vi "set_config_cluster.vi"(8 "error in (no error)":errorcluster, 10 "config cluster variant":variant, 11 "LightSourceDL090909Filament in":refnum<class "LightSourceDL090909Filament.lvclass">) -> (0 "error out":errorcluster, 3 "LightSourceDL090909Filament out":refnum<class "LightSourceDL090909Filament.lvclass">)   [LabVIEW 2010, in "LightSourceDL090909Filament.lvclass"]
uses:
  LightSourceDL090909Filament.lvclass
  LightSourceDL090909Filament.lvclass/LightSourceDL090909Filament.ctl
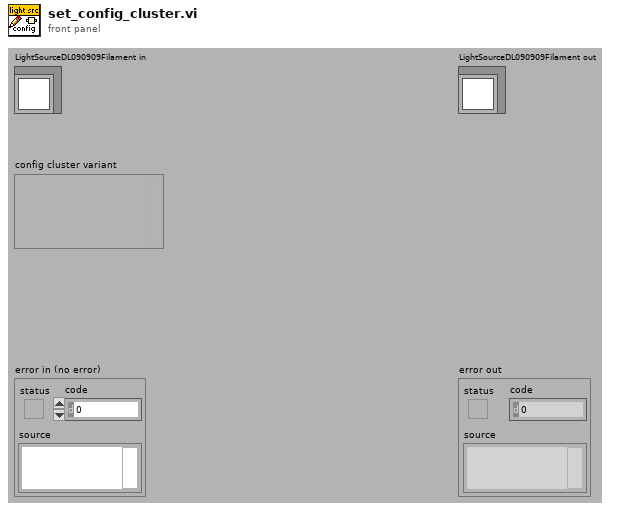
[diagram p1: front panel]
types:
  T1 = typedef "LightSourceDL090909Filament.lvclass/config_data_cluster.ctl" = cluster{"LSID":T2, "manufacturer specification":T3, "type":T4}
  T2 = typedef "LSID_cluster.ctl" = cluster{"identifier":string, "revision":i32}
  T3 = typedef "GenericComponent.lvclass/manufacturer_specification_cluster.ctl" = cluster{"manufacturer":string, "model":string, "serial number":string, "lot number":string}
  T4 = typedef "LightSourceDL090909Filament.lvclass/type_enum.ctl" = enum16{"Incandescent", "Halogen", "Unknown"}
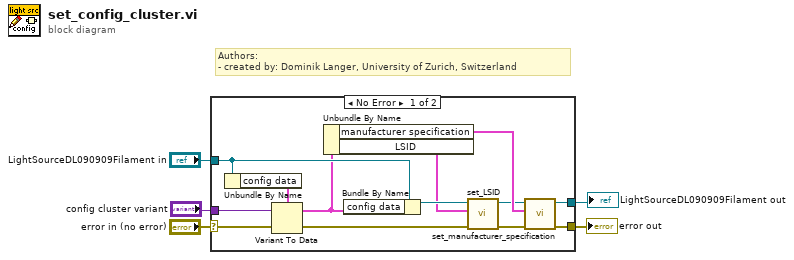
[diagram p0: block diagram]
diagram:
  # "Authors: \n- created by: Dominik Langer, University of Zurich, Switzerland"
  n1 = case shown="No Error" "error in (no error)" {
    selector: "error in (no error)" -> [w13 w20]
    tunnel: [w16 w20] -> w5
    tunnel: [w15 w19] -> w1
    tunnel: "LightSourceDL090909Filament in" -> [w12 w19]
    tunnel: "config cluster variant" -> [w14 _]
    frame No Error {
      n2 = Unbundle By Name(w12) -> ("config data"=w17:T1)
      n3 = Variant To Data(error in=w13, Variant=w14, type=w17) -> (error out=w18:errorcluster, data=w11:T1)
      n4 = Unbundle By Name(w11) -> ("manufacturer specification"=w8:T3, "LSID"=w9:T2)
      n5 = Bundle By Name(cluster=w12, "config data"=w11) -> (w10:refnum<class "LightSourceDL090909Filament.lvclass">)
      n6 = call-dynamic "set_LSID.vi"("error in (no error)"=w18, "LSID"=w9, "GenericPlugin in"=w10) -> ("error out"=w7:errorcluster, "GenericPlugin out"=w6:refnum<class "LightSourceDL090909Filament.lvclass">)  [unwired: 7 in]
      n7 = call-dynamic "set_manufacturer_specification.vi"("error in (no error)"=w7, "manufacturer specification"=w8, "GenericPlugin in"=w6) -> ("error out"=w16:errorcluster, "GenericPlugin out"=w15:refnum<class "LightSourceDL090909Filament.lvclass">)  [unwired: 7 in]
    }
    frame Error {
    }
  }
  "error out" <- w5
  "LightSourceDL090909Filament out" <- w1
